vi "FTW-ProjectItemManager-Read.vi"(0 "Project Item Manager":refnum<class "FTW-ProjectItemManager.lvclass">, 5 "Directive":string, 7 "Default Value":string="NULL", 11 "error in":errorcluster) -> (4 "Project Item Manager out":refnum<class "FTW-ProjectItemManager.lvclass">, 8 "Value":string, 15 "error out":errorcluster)   [LabVIEW 2012, in "FTW-ProjectItemManager.lvclass"]
uses:
  FTW-ProjectItemManager.lvclass
  FTW-ProjectItemManager.lvclass/FTW-ProjectItemManager.ctl
panel:
  # "Inputs"
  # "Outputs"
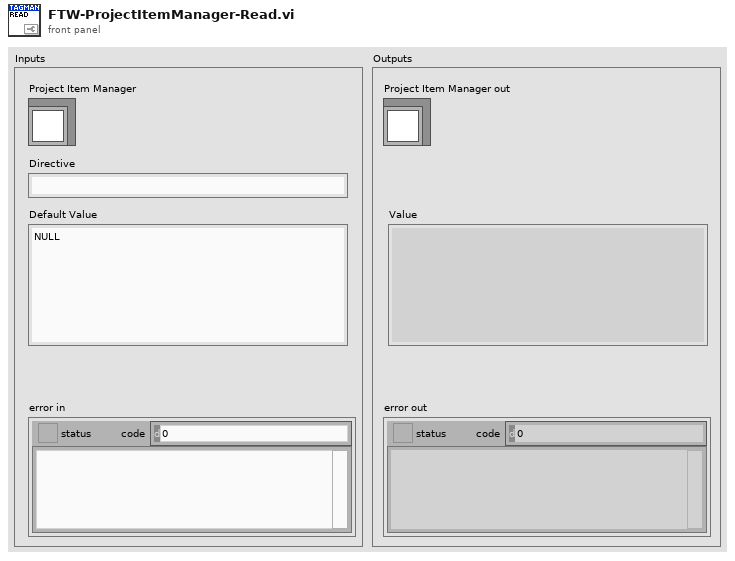
[diagram p1: front panel]
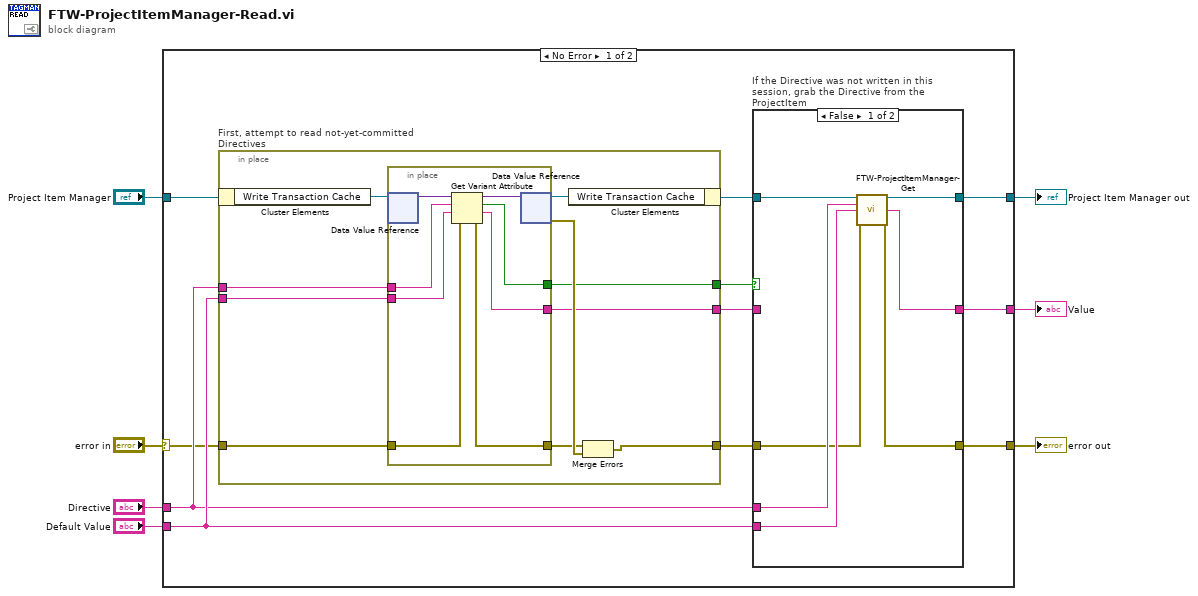
[diagram p0: block diagram]
diagram:
  n1 = case shown="No Error" "error in" {
    selector: "error in" -> [w11 w49]
    tunnel: [w16 w49] -> w7
    tunnel: [w17 w48] -> w5
    tunnel: "Project Item Manager" -> [w15 w48]
    tunnel: "Directive" -> [w12 _]
    tunnel: "Default Value" -> [w13 w47]
    tunnel: [w18 w47] -> w1
    frame No Error {
      n2 = in-place "First, attempt to read not-yet-committed Directives" {
        in-place-border: w11 -> [w38]
        in-place-border: [w31] -> w10
        in-place-border: w12 -> [w37]
        in-place-border: w13 -> [w36]
        in-place-border: [w30] -> w9
        in-place-border: [w29] -> w8
        n3 = in-place-cluster #1(w15) -> ("Write Transaction Cache"=w35:refnum<data-value>)
        n4 = in-place {
          in-place-border: w38 -> [w46]
          in-place-border: [w45] -> w32
          in-place-border: w37 -> [w44]
          in-place-border: w36 -> [w43]
          in-place-border: [w40] -> w30
          in-place-border: [w39] -> w29
          n5 = in-place-dvr #2(w35) -> (w42:variant)  [unwired: 1 out]
          n6 = Get Variant Attribute(Variant=w42, name=w44, default value (empty Variant)=w43, error in=w46) -> (duplicate Variant=w41:variant, found=w40:bool, value=w39:string, error out=w45:errorcluster)
          n7 = in-place-dvr #2(w41) -> (w34:refnum<data-value>, w33:errorcluster)
        }
        n8 = in-place-cluster #1("Write Transaction Cache"=w34) -> (w14:refnum<class "FTW-ProjectItemManager.lvclass">)
        n9 = Merge Errors(w32, w33) -> (w31:errorcluster)
      }
      n10 = case "If the Directive was not written in this\nsession, grab the Directive from the ProjectItem" shown="False" w9 {
        tunnel: [w25 w27] -> w18
        tunnel: [w19 w28] -> w17
        tunnel: [w24 w26] -> w16
        tunnel: w14 -> [w20 w28]
        tunnel: w13 -> [w22 _]
        tunnel: w12 -> [w23 _]
        tunnel: w10 -> [w21 w26]
        tunnel: w8 -> [_ w27]
        frame False {
          n11 = call "FTW-ProjectItemManager-Get.vi"("Project Item Manager"=w20, "Tag"=w23, "Default Value"=w22, "error in"=w21) -> ("Project Item Manager out"=w19:refnum<class "FTW-ProjectItemManager.lvclass">, "Value"=w25:string, "error out"=w24:errorcluster)  [unwired: 9 in]
        }
        frame True {
        }
      }
    }
    frame Error {
    }
  }
  "error out" <- w7
  "Project Item Manager out" <- w5
  "Value" <- w1
